vi "SCLN_ExampleOneClientForParser.vi"() -> ()   [LabVIEW 2015]
uses:
  SCLN_RW_Select.ctl
panel:
  in  "Send":bool
  out "SRV1":errorcluster={"status"=TRUE, "code"=7, "source"="File/Directory Info in Open Config Data.vi->SCLN_ReadConfig.vi->SCLN_InitClient.vi->SCLN_ExampleOneClient.vi"}
  out "Connected 1":bool
  out "Max 1":i32
  out "Loop 1":u32(graph)
  in  "stop":bool
  out "Error 1":errorcluster
  out "Response 1":string
  in  "Command 1":string="sdkfjh qoiwdu wyt op9ei pq9wei n"
  in  "Config Filename":path=path "C:/soar/comm/SCLN/config/soar_comms.cfg"
  # "This VI is the client side of SCLN_ExampleOneServerWithParser.vi.\nReads the command typed in Command 1, after you press SEND.\nThe legal commands for the parser are:\ndate\ntime\npower\ntemperature"
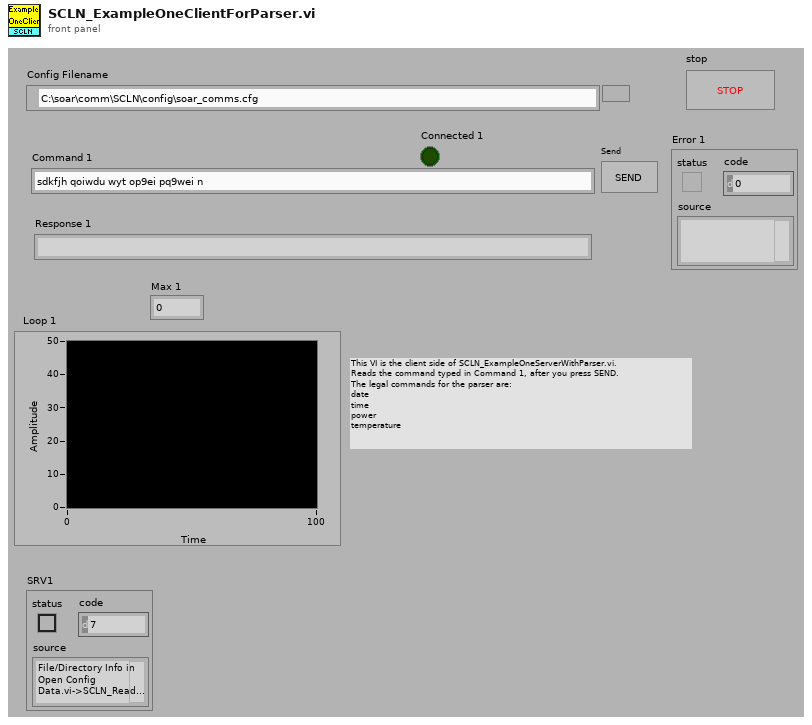
[diagram p1: front panel]
types:
  T1 = typedef "SCLN_RW_Select.ctl" = enum16{"Read", "Write"}
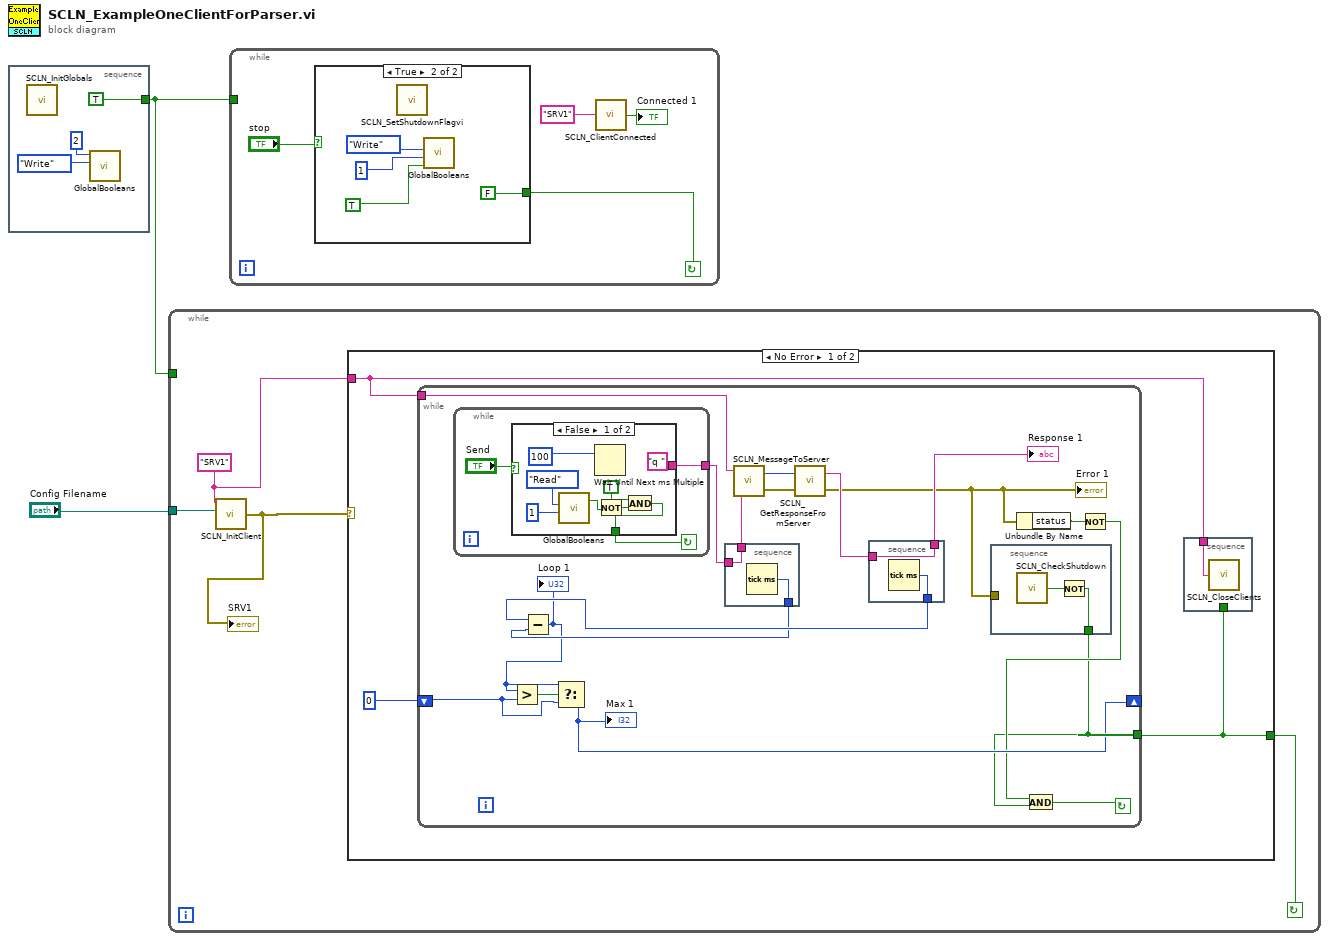
[diagram p0: block diagram]
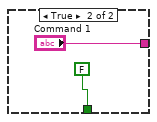
[diagram p2: hidden frame]
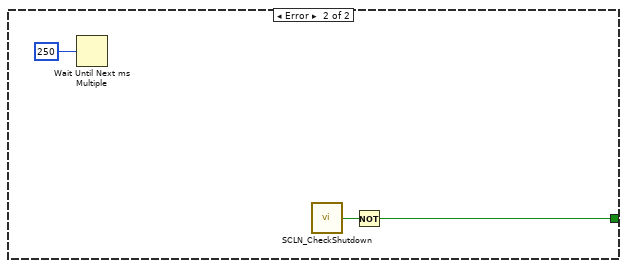
[diagram p3: hidden frame]
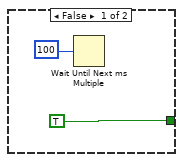
[diagram p4: hidden frame]
diagram:
  n1 = stacked-sequence {
    tunnel: [TRUE] -> w1
    frame #0 {
      n2 = call "SCLN_InitGlobals.vi"() -> ()  [unwired: 1 in]
      n3 = call "GlobalBooleans.vi"("Operation"=SCLN_RW_Select."Write" ("GBL_RW"), "Number of Elements"=2) -> ()  [unwired: 2 in, 2 out]
    }
  }
  n4 = while {
    tunnel: "Config Filename" -> [w9]
    tunnel: w1 -> [_]
    stop <- w8 continue-if-true
    w7 = "SRV1"
    n5 = call "SCLN_InitClient.vi"("Config File Name"=w9, "Server Name"=w7) -> ("error out"=w6:errorcluster)  [unwired: 2 in]
    "SRV1" <- w6
    n6 = case shown="No Error" w6 {
      tunnel: [w11 w51] -> w8
      tunnel: w7 -> [w10 _]
      frame No Error {
        n7 = while {
          shift-right: [w25] -> _
          shift-left: 0 -> [w27]
          tunnel: [w21] -> w11
          tunnel: w10 -> [w20]
          stop <- w22 continue-if-true
          n8 = while {
            tunnel: [w34] -> w16
            stop <- w32 continue-if-true
            n9 = case shown="False" "Send" {
              tunnel: ["q " "Command 1"] -> w34
              tunnel: [w35 FALSE] -> w32
              frame False {
                n10 = call "GlobalBooleans.vi"("Element"=1, "Operation"=SCLN_RW_Select."Read" ("GBL_RW")) -> ("Read Value"=w38:bool)  [unwired: 2 in, 1 out]
                n11 = Wait Until Next ms Multiple(millisecond multiple=100) -> ()  [unwired: 1 out]
                n12 = Not(x=w38) -> (.not. x?=w39:bool)
                n13 = And(x=TRUE, y=w39) -> (x .and. y?=w35:bool)
              }
              frame True {
              }
            }
          }
          n14 = stacked-sequence {
            tunnel: [w50] -> w29
            tunnel: w16 -> [w49]
            tunnel: [w49] -> w15
            frame #0 {
              n15 = Tick Count (ms)() -> (millisecond timer value=w50:u32)
            }
          }
          n16 = call "SCLN_MessageToServer.vi"("Message"=w15, "Server Name"=w20) -> ("error out"=w19:errorcluster, "Index for Response"=w17:i32)  [unwired: 1 in]
          n17 = call "SCLN_GetResponseFromServer.vi"("error in (no error)"=w19, "Index for Response"=w17) -> ("error out"=w14:errorcluster, "Message"=w18:string)
          "Error 1" <- w14
          n18 = stacked-sequence {
            tunnel: w18 -> [w48]
            tunnel: [w48] -> w31
            tunnel: [w47] -> w30
            frame #0 {
              n19 = Tick Count (ms)() -> (millisecond timer value=w47:u32)
            }
          }
          "Response 1" <- w31
          n20 = Subtract(x=w30, y=w29) -> (x-y=w26:u32)
          "Loop 1" <- w26
          n21 = Greater?(x=w26, y=w27) -> (0:w28:bool)
          n22 = Select(t=w26, s=w28, f=w27) -> (s? t:f=w25:u32)
          "Max 1" <- w25
          n23 = stacked-sequence {
            tunnel: [w45] -> w21
            tunnel: w14 -> [_]
            frame #0 {
              n24 = call "SCLN_CheckShutdown.vi"() -> ("Shutdown"=w46:bool)
              n25 = Not(x=w46) -> (.not. x?=w45:bool)
            }
          }
          n26 = Unbundle By Name(w14) -> ("status"=w24:bool)
          n27 = Not(x=w24) -> (.not. x?=w23:bool)
          n28 = And(x=w23, y=w21) -> (x .and. y?=w22:bool)
        }
        n29 = stacked-sequence {
          tunnel: w11 -> [_]
          tunnel: w10 -> [w13]
          frame #0 {
            n30 = call "SCLN_CloseClients.vi"("Server Name"=w13) -> ()
          }
        }
      }
      frame Error {
        n31 = Wait Until Next ms Multiple(millisecond multiple=250) -> ()  [unwired: 1 out]
        n32 = call "SCLN_CheckShutdown.vi"() -> ("Shutdown"=w53:bool)
        n33 = Not(x=w53) -> (.not. x?=w51:bool)
      }
    }
  }
  n34 = while {
    tunnel: w1 -> [_]
    stop <- w56 continue-if-true
    n35 = case shown="True" "stop" {
      tunnel: [TRUE FALSE] -> w56
      frame False {
        n36 = Wait Until Next ms Multiple(millisecond multiple=100) -> ()  [unwired: 1 out]
      }
      frame True {
        n37 = call "SCLN_SetShutdownFlagvi.vi"() -> ()  [unwired: 1 in]
        n38 = call "GlobalBooleans.vi"("Write Value"=TRUE, "Element"=1, "Operation"=SCLN_RW_Select."Write" ("GBL_RW")) -> ()  [unwired: 1 in, 2 out]
      }
    }
    n39 = call "SCLN_ClientConnected.vi"("Server Name"="SRV1") -> ("Connected"=→"Connected 1":bool)
  }
